vi "Get_File_Info_Listing.vi"(0 "path":path) -> (1 "Path":path[](array[path]), 2 "Last Mod":timestamp[](array[timestamp]), 3 "Size":i64[](array[numeric]))   [LabVIEW 2011]
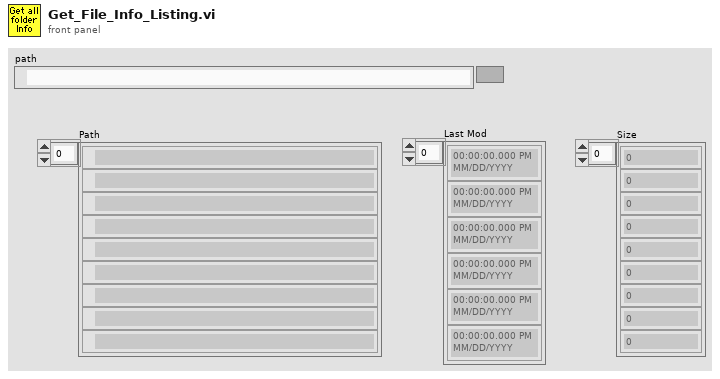
[diagram p1: front panel]
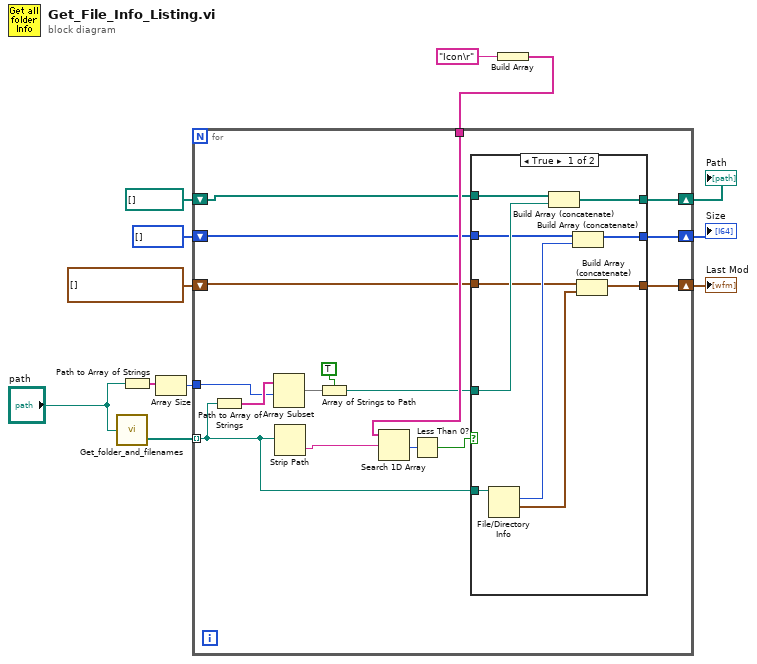
[diagram p0: block diagram]
diagram:
  n1 = call "Get_folder_and_filenames.vi"("file path (dialog if empty)"="path") -> ("Files"=w8:path[])  [unwired: 1 out]
  n2 = Path to Array of Strings(0:"path") -> (2:w9:string[])  [unwired: 1 out]
  n3 = Array Size(array=w9) -> (size(s)=w10:i32)
  n4 = Build Array("Icon\r") -> (w12:string[])
  n5 = for {
    tunnel: w8 -> [w20] mode=indexing
    tunnel: w10 -> [w27]
    shift-right: [w17] -> w1
    shift-left: path[] [] -> [w19]
    tunnel: w12 -> [w25]
    shift-right: [w15] -> w2
    shift-left: i64[] [] -> [w16]
    shift-right: [w13] -> w3
    shift-left: timestamp[] [] -> [w14]
    n6 = Path to Array of Strings(0:w20) -> (2:w28:string[])  [unwired: 1 out]
    n7 = Array Subset(array=w28, index=w27) -> (w23:string[])  [unwired: 1 in]
    n8 = Strip Path(path=w20) -> (name=w26:string)  [unwired: 1 out]
    n9 = Array of Strings to Path(0:w23, 1:TRUE ("relative")) -> (2:w18:path)
    n10 = Search 1D Array(1D array=w25, element=w26) -> (index of element=w24:i32)  [unwired: 1 out]
    n11 = Less Than 0?(x=w24) -> (x < 0?=w21:bool)
    n12 = case shown="True" w21 {
      tunnel: w20 -> [w38 _]
      tunnel: w19 -> [w37 w41]
      tunnel: w18 -> [w36 _]
      tunnel: [w35 w41] -> w17
      tunnel: w16 -> [w32 w40]
      tunnel: [w31 w40] -> w15
      tunnel: w14 -> [w30 w39]
      tunnel: [w29 w39] -> w13
      frame True {
        n13 = File/Directory Info(path=w38) -> (size=w33:i64, last mod=w34:timestamp)  [unwired: 1 in, 5 out]
        n14 = Build Array (concatenate)(w37, w36) -> (w35:path[])
        n15 = Build Array (concatenate)(w32, w33) -> (w31:i64[])
        n16 = Build Array (concatenate)(w30, w34) -> (w29:timestamp[])
      }
      frame False {
      }
    }
  }
  "Last Mod" <- w3
  "Size" <- w2
  "Path" <- w1
